vi "Get Name, Value, URL.vi"(8 "error in (no error)":errorcluster, 11 "Refnum in":refnum<k20>) -> (0 "error out":errorcluster, 1 "URL":string, 2 "Type":string, 3 "Name":string)   [LabVIEW 2016]
uses:
  <vilib>/xml/Close Reference(NNMap).vi
  <vilib>/xml/Close Reference(Node).vi
  <resource>/objmgr/DOMUserDefRef.rc
  <vilib>/xml/NI_XML.lvlib
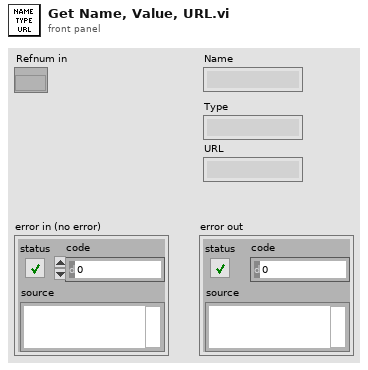
[diagram p1: front panel]
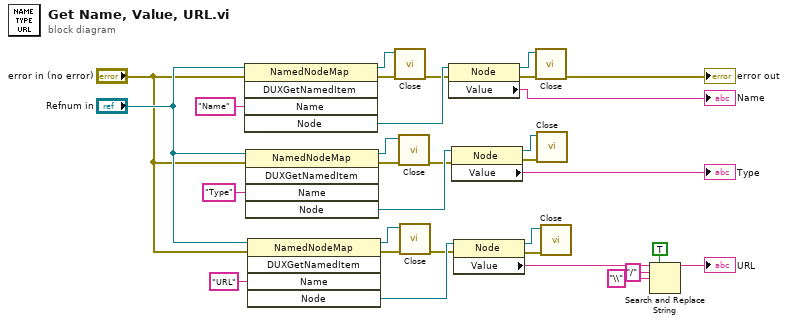
[diagram p0: block diagram]
diagram:
  n1 = invoke class="NamedNodeMap" method="DUXGetNamedItem"(reference="Refnum in", error in="error in (no error)", "Name"="Name") -> (reference out=w8:refnum<k20>, error out=w16:errorcluster, "Node"=w30:refnum<k20>)  [unwired: 2 in, 2 out]
  n2 = invoke class="NamedNodeMap" method="DUXGetNamedItem"(reference="Refnum in", error in="error in (no error)", "Name"="Type") -> (reference out=w9:refnum<k20>, error out=w11:errorcluster, "Node"=w24:refnum<k20>)  [unwired: 2 in, 2 out]
  n3 = invoke class="NamedNodeMap" method="DUXGetNamedItem"(reference="Refnum in", error in="error in (no error)", "Name"="URL") -> (reference out=w14:refnum<k20>, error out=w13:errorcluster, "Node"=w23:refnum<k20>)  [unwired: 2 in, 2 out]
  n4 = call-poly <vilib>:"Close.vi"("error in (no error)"=w16, "named node map"=w8) -> ("error out"=w15:errorcluster)  [unwired: 7 in]
  n5 = call-poly <vilib>:"Close.vi"("error in (no error)"=w11, "named node map"=w9) -> ("error out"=w10:errorcluster)  [unwired: 7 in]
  n6 = call-poly <vilib>:"Close.vi"("error in (no error)"=w13, "named node map"=w14) -> ("error out"=w12:errorcluster)  [unwired: 7 in]
  n7 = property class="Node"(reference=w30, error in=w15) -> (reference out=w7:refnum<k20>, error out=w6:errorcluster, "Value"=→"Name":string)
  n8 = property class="Node"(reference=w24, error in=w10) -> (reference out=w3:refnum<k20>, error out=w4:errorcluster, "Value"=→"Type":string)
  n9 = property class="Node"(reference=w23, error in=w12) -> (reference out=w2:refnum<k20>, error out=w1:errorcluster, "Value"=w21:string)
  n10 = call-poly <vilib>:"Close.vi"("error in (no error)"=w6, "node"=w7) -> ("error out"=→"error out":errorcluster)  [unwired: 7 in]
  n11 = call-poly <vilib>:"Close.vi"("error in (no error)"=w4, "node"=w3) -> ()  [unwired: 7 in, 1 out]
  n12 = call-poly <vilib>:"Close.vi"("error in (no error)"=w1, "node"=w2) -> ()  [unwired: 7 in, 1 out]
  n13 = Search and Replace String(replace all?=TRUE ("replace all? (F)"), input string=w21, search string="/", replace string="\\" ("replace string (\"\")")) -> (result string=→"URL":string)  [unwired: 4 in, 3 out]
